vi "DrawHexagonalLattice.vi"(10 "Size":i32, 11 "Lattice Constant":dbl) -> (3 "E1":dbl[][](array[numeric]))   [LabVIEW 2017]
uses:
  <vilib>/imath/engines/lvmath2/RunTimeEngine/RangeToken/NIMS_Range.vi
  <instcachedir>/0/NIMS_Range_8C005833F4504FD4A29AA23D6150121A.lvgen/NIMS_Range_8C005833F4504FD4A29AA23D6150121A_001.vi
  <vilib>/imath/engines/lvmath2/RunTimeEngine/BuiltInFunctions/meshgrid2d/NIMS_meshgrid2d(V).vi
  <instcachedir>/0/NIMS_meshgrid2d(V)_B267DDA9BCD34B1A861DA092682A58DE.lvgen/NIMS_meshgrid2d(V)_B267DDA9BCD34B1A861DA092682A58DE_002.vi
  <vilib>/imathl/engines/lvmath/Functions/Error Handling/Create Error.vi
  <vilib>/imath/engines/lvmath2/RunTimeEngine/IndexRead/NIMS M($).vi
  <instcachedir>/0/NIMS M($)_82D1177398184AFB96A6AFB63C3C3F57.lvgen/NIMS M($)_82D1177398184AFB96A6AFB63C3C3F57_000.vi
  <vilib>/imath/engines/lvmath2/RunTimeEngine/ArithmeticOperatorToken/NIMS_ArithmeticOperator_plus.vi
  <instcachedir>/0/NIMS_ArithmeticOperator_plus_83A06A2F5B774300BF206C47F5885884.lvgen/NIMS_ArithmeticOperator_plus_83A06A2F5B774300BF206C47F5885884_004.vi
  <vilib>/imath/engines/lvmath2/RunTimeEngine/RowToken/NIMS_RowToken_CV_CV.vi
  <instcachedir>/0/NIMS_RowToken_CV_CV_289591C7021745DEB083F10AE9949B55.lvgen/NIMS_RowToken_CV_CV_289591C7021745DEB083F10AE9949B55_000.vi
  <vilib>/imath/engines/lvmath2/RunTimeEngine/ErrorHandling/NIMS_Create Error From Enums.vi
  <vilib>/imath/engines/lvmath2/RunTimeEngine/BuiltInFunctions/eps/NIMS_eps.vi
  <vilib>/imath/engines/lvmath2/RunTimeEngine/IndexRead/NIMS M($,S).vi
  <instcachedir>/0/NIMS M($,S)_3E5749BBB62E49528D4765A77F1F6D98.lvgen/NIMS M($,S)_3E5749BBB62E49528D4765A77F1F6D98_000.vi
  <vilib>/imath/engines/lvmath2/RunTimeEngine/BuiltInFunctions/abs/NIMS_abs(signed).vi
  <instcachedir>/0/NIMS_abs(signed)_C4FCB8E6058B49B797C7C8D53CA5F6EC.lvgen/NIMS_abs(signed)_C4FCB8E6058B49B797C7C8D53CA5F6EC_001.vi
  <vilib>/imath/engines/lvmath2/RunTimeEngine/VariableToken/Support/NIMS_Vector Boolean Index to I32 Index.vi
  <vilib>/imath/engines/lvmath2/RunTimeEngine/IndexReplace/NIMS M(V,$)=M.vi
  <instcachedir>/0/NIMS M(V,$)=M_013E6DB4A5AE4B1980728FF3E9F70CE5.lvgen/NIMS M(V,$)=M_013E6DB4A5AE4B1980728FF3E9F70CE5_003.vi
  <vilib>/imath/engines/lvmath2/RunTimeEngine/NodeEndStatement/NIMS_NodeEndStatement_Output.vi
  <instcachedir>/0/NIMS_NodeEndStatement_Output_53EC0D466D134D7ABD903AC30B43404B.lvgen/NIMS_NodeEndStatement_Output_53EC0D466D134D7ABD903AC30B43404B_002.vi
  <vilib>/imath/engines/lvmath2/RunTimeEngine/ErrorHandling/NIMS_Finalize Error.vi
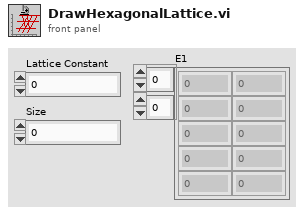
[diagram p1: front panel]
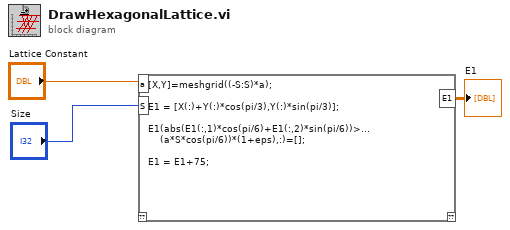
[diagram p0: block diagram]
diagram:
  n1 = mathscript code="[X,Y]=meshgrid((-S:S)*a);\n\nE1 = [X(:)+Y(:)*cos(pi/3),Y(:)*sin(pi/3)];\n\nE1(abs(E1(:,1)*cos(pi/6)+E1(:,2)*sin(pi/6))>...\n    (a*S*cos(pi/6))*(1+eps),:)=[];\n\nE1 = E1+75;"("a"="Lattice Constant", "S"="Size") -> ("E1"=→"E1":dbl[][])  [unwired: 1 in, 1 out]
